vi "getDaySecs.vi"() -> (0 "x+y":dbl)   [LabVIEW 2015]
panel:
  out "date/time string":string="15:37"
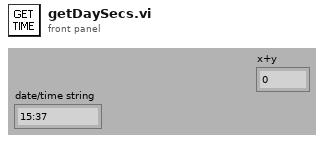
[diagram p1: front panel]
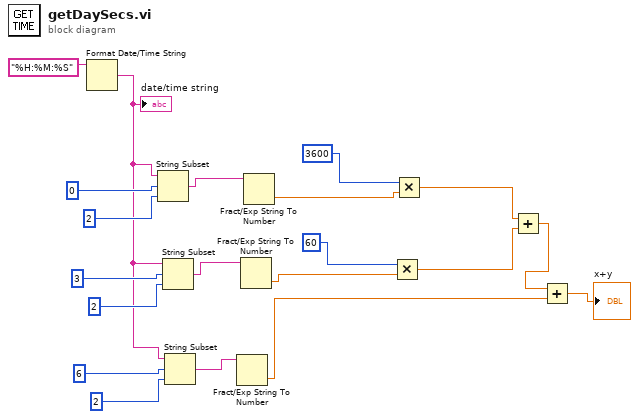
[diagram p0: block diagram]
diagram:
  n1 = Format Date/Time String(time format string (%c)="%H:%M:%S") -> (date/time string=w13:string)  [unwired: 2 in]
  "date/time string" <- w13
  n2 = String Subset(string=w13, offset (0)=0, length (rest)=2) -> (substring=w12:string)
  n3 = String Subset(string=w13, offset (0)=3, length (rest)=2) -> (substring=w10:string)
  n4 = String Subset(string=w13, offset (0)=6, length (rest)=2) -> (substring=w11:string)
  n5 = Fract/Exp String To Number(string=w11) -> (number=w3:dbl)  [unwired: 3 in, 1 out]
  n6 = Fract/Exp String To Number(string=w10) -> (number=w8:dbl)  [unwired: 3 in, 1 out]
  n7 = Fract/Exp String To Number(string=w12) -> (number=w7:dbl)  [unwired: 3 in, 1 out]
  n8 = Multiply(x=60, y=w8) -> (x*y=w4:dbl)
  n9 = Multiply(x=3600, y=w7) -> (x*y=w5:dbl)
  n10 = Add(x=w5, y=w4) -> (x+y=w2:dbl)
  n11 = Add(x=w2, y=w3) -> (x+y=→"x+y":dbl)
